vi "ParseUpdatePassword.vi"(8 "error in (no error)":errorcluster, 11 "body":variant) -> (0 "error out":errorcluster, 2 "Update Password":T1)   [LabVIEW 2017, in "ServerComm.lvlib"]
uses:
  <vilib>/addons/InsightCM/Devices/Shared/Common/ServerComm/ServerComm.lvlib
  <vilib>/addons/InsightCM/Devices/Shared/Common/ServerComm/controls/UpdatePassword.ctl
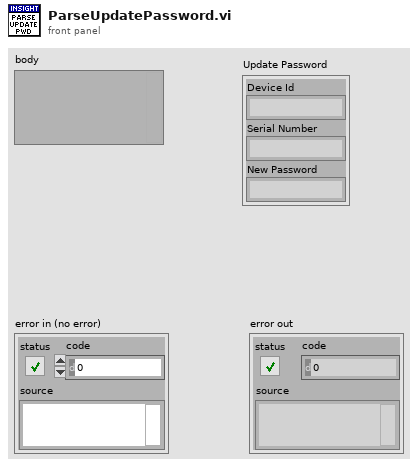
[diagram p1: front panel]
types:
  T1 = typedef "ServerComm.lvlib/UpdatePassword.ctl" = cluster{"Device Id":string, "Serial Number":string, "New Password":string}
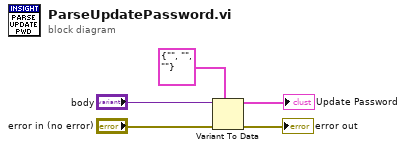
[diagram p0: block diagram]
diagram:
  n1 = Variant To Data(error in="error in (no error)", type=T1 {"Device Id"="", "Serial Number"="", "New Password"=""} ("Update Password 2"), Variant="body") -> (data=→"Update Password":T1, error out=→"error out":errorcluster)
